vi "Box_Expand_or_Contract.vi"(1 "Rectangle in":T1, 2 "Expand/Contract":i32) -> (0 "Rectangle out":T1)   [LabVIEW 2018, in "Cage Diagram.lvlib"]
uses:
  Cage Diagram.lvlib
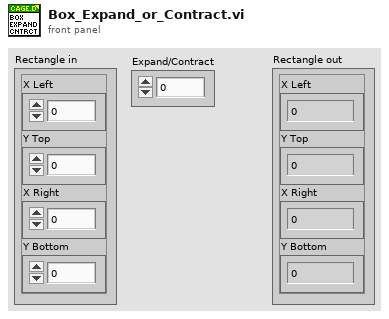
[diagram p1: front panel]
types:
  T1 = cluster{"X Left":i32, "Y Top":i32, "X Right":i32, "Y Bottom":i32}
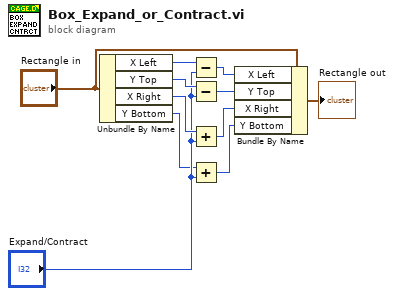
[diagram p0: block diagram]
diagram:
  n1 = Unbundle By Name("Rectangle in") -> ("X Left"=w10:i32, "Y Top"=w9:i32, "X Right"=w8:i32, "Y Bottom"=w6:i32)
  n2 = Subtract(x=w10, y="Expand/Contract") -> (x-y=w5:i32)
  n3 = Subtract(x=w9, y="Expand/Contract") -> (x-y=w4:i32)
  n4 = Add(x=w8, y="Expand/Contract") -> (x+y=w3:i32)
  n5 = Add(x=w6, y="Expand/Contract") -> (x+y=w2:i32)
  n6 = Bundle By Name(cluster="Rectangle in", "X Left"=w5, "Y Top"=w4, "X Right"=w3, "Y Bottom"=w2) -> (→"Rectangle out":T1)
